vi "load_start.vi"(8 "error in (no error)":errorcluster, 10 "start":i16, 11 "Instrument in":refnum<class "Instrument.lvclass">) -> (0 "error out":errorcluster, 3 "Instrument out":refnum<class "Instrument.lvclass">)   [LabVIEW 2019, in "Instrument.lvclass"]
uses:
  Instrument.lvclass
  Instrument.lvclass/Instrument.ctl
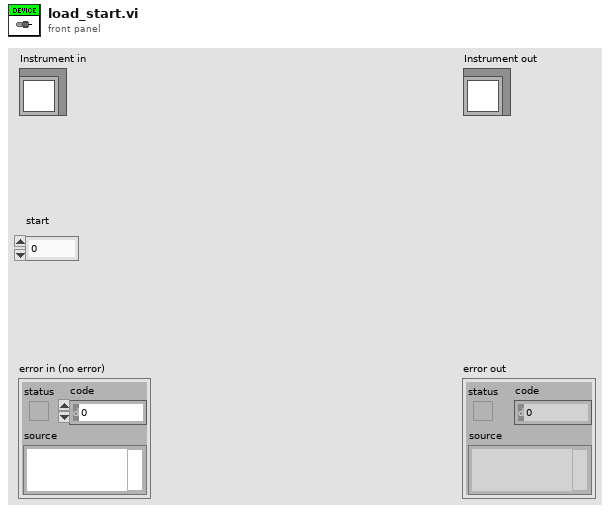
[diagram p1: front panel]
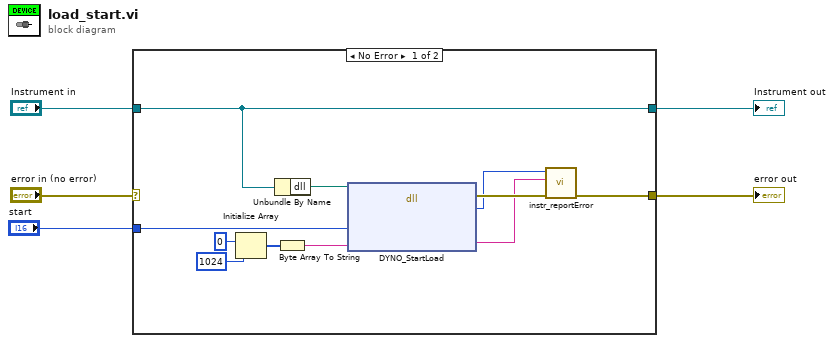
[diagram p0: block diagram]
diagram:
  n1 = case shown="No Error" "error in (no error)" {
    selector: "error in (no error)" -> [_ w18]
    tunnel: [w11 w18] -> w4
    tunnel: [w16 w17] -> w2
    tunnel: "Instrument in" -> [w16 w17]
    tunnel: "start" -> [w6 _]
    frame No Error {
      n2 = Initialize Array(u8 0 ("element"), 1024 ("dimension size")) -> (w8:u8[])
      n3 = Unbundle By Name(w16) -> ("dll"=w15:path)
      n4 = Byte Array To String(unsigned byte array=w8) -> (string=w7:string)
      n5 = dll-call lib="C:/Dev/22KW-Dyno/software/data/DynoAPI.dll" fn="DYNO_StartLoad"(path in=w15, "start"=w6, "errorMsg"=w7) -> (error out=w14:errorcluster, "return type"=w13:i32, "errorMsg"=w12:string)  [unwired: 3 in, 1 out]
      n6 = call "instr_reportError.vi"("error in (no error)"=w14, "errorMsg"=w12, "return type"=w13) -> ("error out"=w11:errorcluster)  [unwired: 8 in]
    }
    frame Error {
    }
  }
  "error out" <- w4
  "Instrument out" <- w2
